vi "Shooting Module.vi"(11 "distance\n(Meters)":dbl(slide) scale=0.0..6.0 scale format="%3d") -> (2 "Magnitude":dbl, 3 "Encoder Degrees":dbl)   [LabVIEW 2013]
panel:
  out "distance\n(Feet)":dbl(slide) scale=0.0..20.0 scale format="%3d"
  out "Shooting Range":bool
  out "RPM":i32
  out "Catapult Move\nAngle":i32
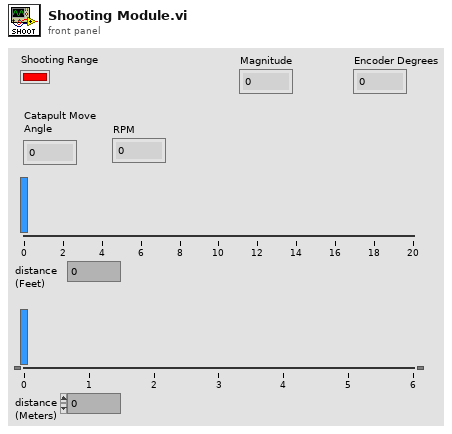
[diagram p1: front panel]
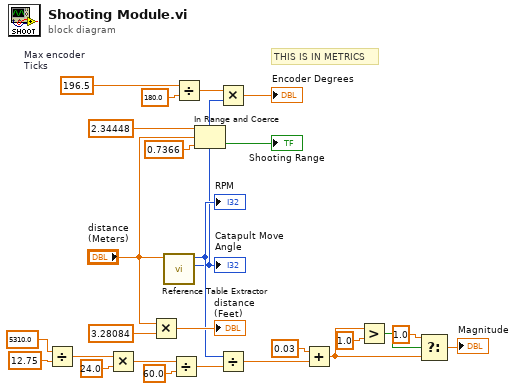
[diagram p0: block diagram]
diagram:
  w1 = 196.5  # Max encoder Ticks
  # "THIS IS IN METRICS"
  n1 = Divide(x=5310.0, y=12.75) -> (x/y=w24:dbl)
  n2 = Multiply(x=w24, y=24.0) -> (x*y=w22:dbl)
  n3 = Multiply(x="distance\n(Meters)", y=3.28084) -> (x*y=→"distance\n(Feet)":dbl)
  n4 = call "Reference Table Extractor.vi"("distance"="distance\n(Meters)") -> ("Catapult Move\nAngle"=w5:i32, "RPM"=w7:i32)  [unwired: 7 in, 2 out]
  "Catapult Move\nAngle" <- w5
  "RPM" <- w7
  n5 = Divide(x=w22, y=60.0) -> (x/y=w16:dbl)
  n6 = Divide(x=w1, y=180.0) -> (x/y=w8:dbl)
  n7 = In Range and Coerce(upper limit=2.34448, x="distance\n(Meters)", lower limit=0.7366 ("y")) -> (In Range?=→"Shooting Range":bool)  [unwired: 1 out]
  n8 = Multiply(x=w8, y=w5) -> (x*y=→"Encoder Degrees":dbl)
  n9 = Divide(x=w7, y=w16) -> (x/y=w4:dbl)
  n10 = Add(x=0.03, y=w4) -> (x+y=w3:dbl)
  n11 = Greater?(x=w3, y=1.0) -> (0:w19:bool)
  n12 = Select(t=1.0, s=w19, f=w3) -> (s? t:f=→"Magnitude":dbl)
